vi "SetParam.vi"(8 "error in (no error)":errorcluster caption="entrée d'erreur (pas d'erreur)", 10 "StratifiedKFold":T1={"n_splits"=5, "shuffle"=FALSE, "random_state"=-1} {"random_state" min=-1}, 11 "StratifiedKFold.lvclass":refnum<class "StratifiedKFold.lvclass">) -> (0 "error out":errorcluster caption="sortie d'erreur", 3 "StratifiedKFold.lvclass":refnum<class "StratifiedKFold.lvclass">)   [LabVIEW 2020, in "StratifiedKFold.lvclass"]
doc: "Set Parameters"
uses:
  StratifiedKFold.lvclass
  StratifiedKFold.lvclass/StratifiedKFold.ctl
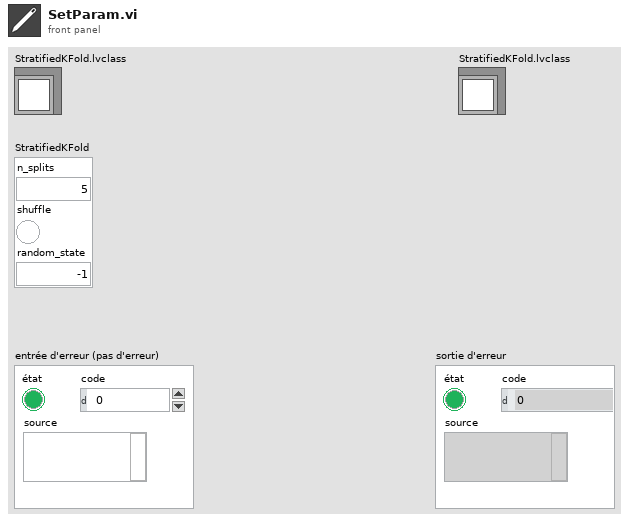
[diagram p1: front panel]
types:
  T1 = cluster{"n_splits":i32, "shuffle":bool, "random_state":i32}
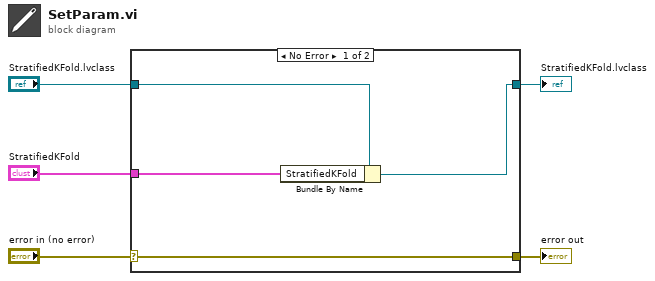
[diagram p0: block diagram]
diagram:
  n1 = case shown="No Error" "error in (no error)" {
    selector: "error in (no error)" -> [w9 w10]
    tunnel: [w9 w10] -> w4
    tunnel: [w7 w11] -> w2
    tunnel: "StratifiedKFold.lvclass" -> [w8 w11]
    tunnel: "StratifiedKFold" -> [w6 _]
    frame No Error {
      n2 = Bundle By Name(cluster=w8, "StratifiedKFold"=w6) -> (w7:refnum<class "StratifiedKFold.lvclass">)
    }
    frame Error {
    }
  }
  "error out" <- w4
  "StratifiedKFold.lvclass" <- w2
